vi "Calibrate.vi"(8 "error in (no error)":errorcluster, 11 "KUKA youBot arm motor in":refnum<class "NI_Robotics_KUKA youBot Arm Motor.lvclass">) -> (0 "error out":errorcluster, 3 "KUKA youBot arm motor out":refnum<class "NI_Robotics_KUKA youBot Arm Motor.lvclass">)   [LabVIEW 2017, in "NI_Robotics_KUKA youBot Host.lvlib" / "NI_Robotics_KUKA youBot Arm Motor.lvclass"]
uses:
  <vilib>/robotics/KUKA youBot/Motor/Arm Motor/NI_Robotics_KUKA youBot Arm Motor.lvclass
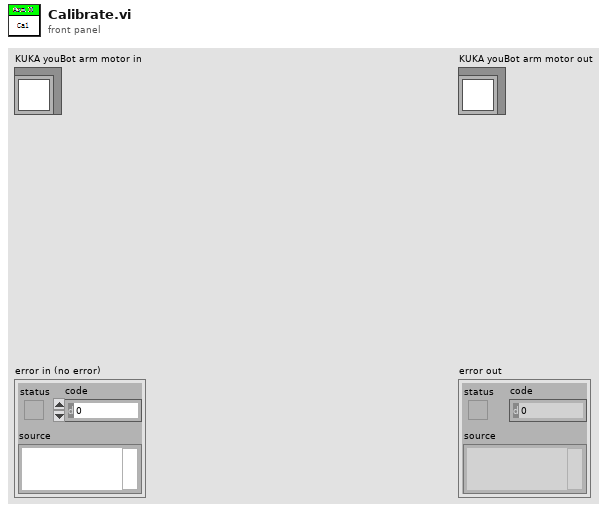
[diagram p1: front panel]
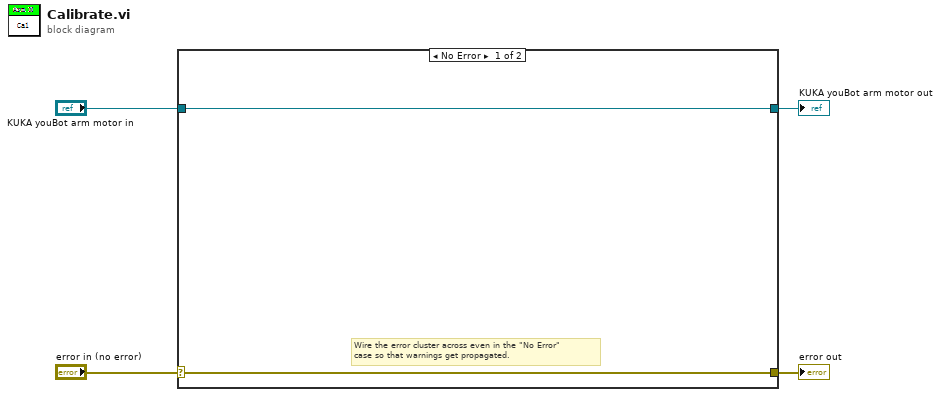
[diagram p0: block diagram]
diagram:
  n1 = case shown="No Error" "error in (no error)" {
    selector: "error in (no error)" -> [w5 w8]
    tunnel: [w5 w8] -> w3
    tunnel: [w6 w7] -> w1
    tunnel: "KUKA youBot arm motor in" -> [w6 w7]
    frame No Error {
      # "Wire the error cluster across even in the \"No Error\"\ncase so that warnings get propagated."
    }
    frame Error {
    }
  }
  "error out" <- w3
  "KUKA youBot arm motor out" <- w1
